vi "SerialMarvinSendGet.vi"(8 "error in (no error)":errorcluster, 9 "Clear Log":bool, 10 "write buffer":string="UA[3]\r\n", 11 "VISA resource name":refnum<visa-resource-name>="COM6") -> (0 "error out":errorcluster, 2 "read buffer":string)   [LabVIEW 2017]
uses:
  <vilib>/Instr/_visa.llb/VISA Configure Serial Port (Instr).vi
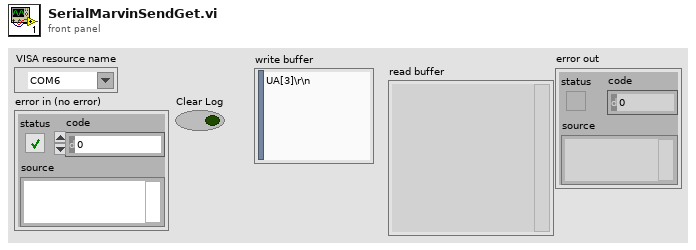
[diagram p1: front panel]
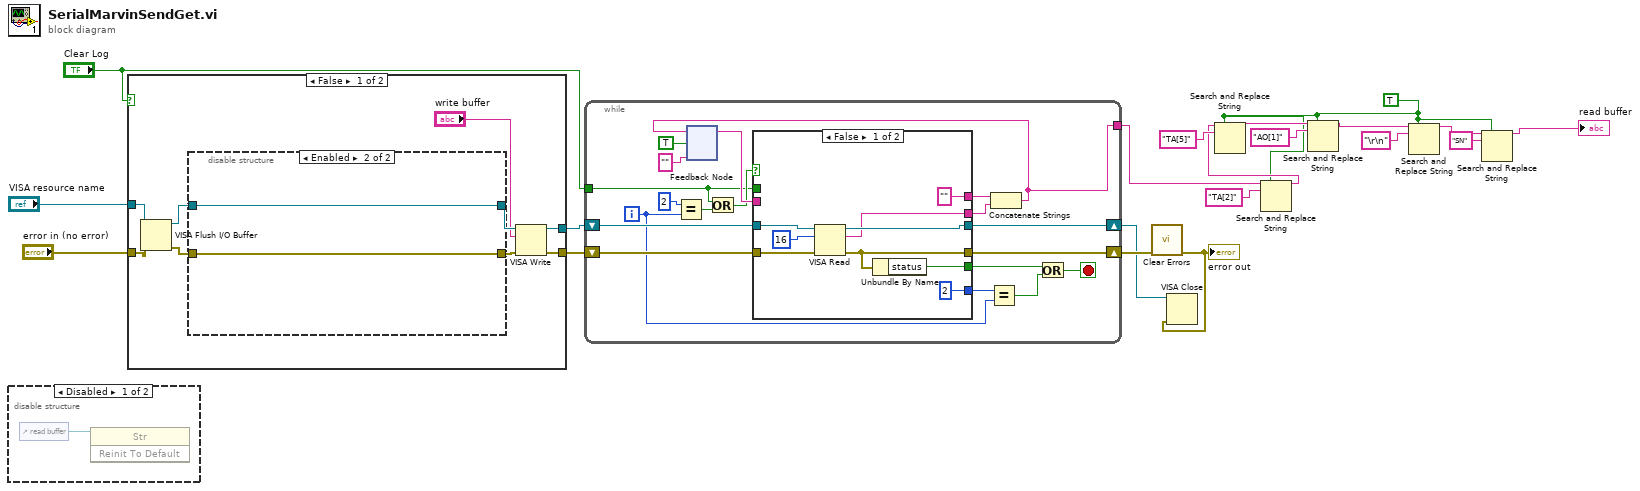
[diagram p0: block diagram]
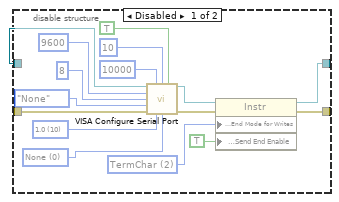
[diagram p3: hidden frame]
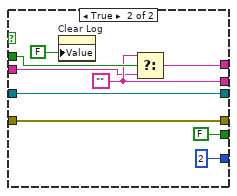
[diagram p5: hidden frame]
diagram:
  w3 = TRUE ("replace all? (F)")
  n1 = disable-structure shown="Disabled" {
    frame Disabled {
      n2 = control-ref of="read buffer"() -> (w21:refnum<vi>)
      n3 = invoke class="Str" method="Reinit To Default"(reference=w21) -> ()  [unwired: 2 in, 3 out]
    }
    frame Enabled {
    }
  }
  n4 = case shown="False" "Clear Log" {
    tunnel: "VISA resource name" -> [w23 w50]
    tunnel: "error in (no error)" -> [w25 w49]
    tunnel: [w28 w50] -> w17
    tunnel: [w27 w49] -> w16
    frame False {
      n5 = VISA Flush I/O Buffer(VISA resource name=w23, error in (no error)=w25) -> (VISA resource name out=w22:refnum<visa-resource-name>, error out=w24:errorcluster)  [unwired: 1 in]
      n6 = disable-structure shown="Enabled" {
        disable-tunnel: w22 -> [w46 w48]
        disable-tunnel: w24 -> [w40 w47]
        disable-tunnel: [w35 w48] -> w29
        disable-tunnel: [w34 w47] -> w30
        frame Disabled {
          w32 = u16 2 items=["None", "LastBit", "TermChar", "Break"] ("Serial Settings:Serial End Mode for Writes")
          w38 = u16 0 items=["None", "XON/XOFF", "RTS/CTS", "XON/XOFF & RTS/CTS", "DTR/DSR", "XON/XOFF & DTR/DSR"] ("flow control (0:none)")
          w39 = u16 10 items=["1.0"=10, "1.5"=15, "2.0"=20] ("stop bits (10: 1 bit)")
          n7 = call-poly "VISA Configure Serial Port"("VISA resource name"=w46, "timeout (10sec)"=u32 10000, "termination char\n(0xA = '\\n' = LF)"=u8 10 ("termination char\n(0xA = '\\n' = LF)"), "Enable Termination\nChar (T)"=TRUE ("Enable Termination\nChar (T)"), "baud rate (9600)"=u32 9600, "data bits (8)"=u16 8, "parity (0:none)"=enum16{"None", "Odd", "Even", "Mark", "Space"}."None", "error in (no error)"=w40, "stop bits (10: 1 bit)"=w39, "flow control (0:none)"=w38) -> ("VISA resource name out"=w36:refnum<visa-resource-name>, "error out"=w37:errorcluster)  [unwired: 4 in]
          n8 = property class="Instr"(reference=w36, error in=w37, "Serial Settings:End Mode for Writes"=w32, "Message Based Settings:Send End Enable"=TRUE) -> (reference out=w35:refnum<visa-resource-name>, error out=w34:errorcluster)
        }
        frame Enabled {
        }
      }
      n9 = VISA Write(VISA resource name=w29, write buffer="write buffer", error in (no error)=w30) -> (VISA resource name out=w28:refnum<visa-resource-name>, error out=w27:errorcluster)  [unwired: 1 out]
    }
    frame True {
    }
  }
  n10 = while {
    shift-right: [w69] -> w2
    shift-left: w17 -> [w65]
    shift-right: [w67] -> w20
    shift-left: w16 -> [w64]
    tunnel: [w51] -> w5
    tunnel: "Clear Log" -> [w56]
    i -> [w60]
    stop <- w52 stop-if-true
    n11 = Equal?(x=2, y=w60) -> (x = y?=w58:bool)
    n12 = feedback #1("") -> (w63:string)
    n13 = Or(x=w56, y=w58) -> (x .or. y?=w57:bool)
    n14 = case shown="False" w57 {
      tunnel: [w78 w87] -> w69
      tunnel: [w77 w81] -> w68
      tunnel: [w75 w86] -> w67
      tunnel: [w74 FALSE ("status")] -> w66
      tunnel: w65 -> [w73 w87]
      tunnel: w64 -> [w72 w86]
      tunnel: w63 -> [_ w80]
      tunnel: ["" w79] -> w62
      tunnel: [2 ("x") 2 ("x")] -> w61
      tunnel: w56 -> [_ w82]
      frame False {
        n15 = VISA Read(VISA resource name=w73, byte count=u32 16, error in (no error)=w72) -> (VISA resource name out=w78:refnum<visa-resource-name>, read buffer=w77:string, error out=w75:errorcluster)  [unwired: 1 out]
        n16 = Unbundle By Name(w75) -> ("status"=w74:bool)
      }
      frame True {
        w81 = ""
        n17 = property on="Clear Log" class="Bool (strict)"("Value"=FALSE ("Clear Log")) -> ()  [unwired: 2 in, 2 out]
        n18 = Select(t=w81, s=w82, f=w80) -> (s? t:f=w79:string)
      }
    }
    n19 = Equal?(x=w61, y=w60) -> (x = y?=w53:bool)
    n20 = Concatenate Strings(w62, w68) -> (w51:string)
    n21 = feedback-in #1(w51, TRUE) -> ()
    n22 = Or(x=w66, y=w53) -> (x .or. y?=w52:bool)
  }
  n23 = call <vilib>:"Clear Errors.vi"("error in (no error)"=w20) -> ("error out"=w1:errorcluster)  [unwired: 5 in, 1 out]
  "error out" <- w1
  n24 = VISA Close(VISA resource name=w2, error in (no error)=w1) -> ()  [unwired: 1 out]
  n25 = Search and Replace String(replace all?=w3, input string=w5, search string="TA[2]" ("substring (\"\")")) -> (result string=w4:string)  [unwired: 5 in, 3 out]
  n26 = Search and Replace String(replace all?=w3, input string=w4, search string="TA[5]" ("substring (\"\")")) -> (result string=w12:string)  [unwired: 5 in, 3 out]
  n27 = Search and Replace String(replace all?=w3, input string=w12, search string="AO[1]" ("substring (\"\")")) -> (result string=w10:string)  [unwired: 5 in, 3 out]
  n28 = Search and Replace String(replace all?=w3, input string=w10, search string="\r\n" ("substring (\"\")")) -> (result string=w9:string)  [unwired: 5 in, 3 out]
  n29 = Search and Replace String(replace all?=w3, input string=w9, search string="SN") -> (result string=→"read buffer":string)  [unwired: 5 in, 3 out]
